vi "lorentzian from circle corners V7.vi"(6 "cursor bracket in":T1={"left"=2044.0881763527054, "right "=2126.7657992565055, "center"=2085.4269878046052, "window"=82.67762290380006, "cursors"=[], "relative"=0, "absolute"=0, "fixed vertical offset"=2421.6740576496672, "vertical offset"=2421.6740576496672, "skew"=2421.6740576496672, "default window frac"=2421.6740576496672, "kind"=enum."fancy", "skew.left"=2.0, "skew.right"=0.0, "Plot ref"=refnum, "wing order"=enum."back"}, 7 "update z(inf)":enum16{"update z(inf)", "do not update z(inf)"}(ring)=enum."do not update z(inf)", 8 "omega map rameters in":T7={"map method"=enum."less trivial", "2:window factor"=1, "left"=3.0, "right"=3.0, "omega"=3.0, "gamma"=3.0, "theta0"=3.0, "use points"=enum."decimated", "z(inf) method"=enum."median"}, 10 "parameters in: center detection":T6={"number of 2D grid points"=200, "# of points in pond"=93, "# of points in window"=4107, "decimation threshold"=1, "normalization factor"=0.005102552585135461, "pond scale factor "=3.0, "normalized z"=[], "decimated z"=[], "decimated omega"=[], "omega in window"=[], "z in window"=[], "data center"=-0.0014901433980738042-0.0014987103874714112i, "inverse"=[], "linear "=[], "omega around"=[], "phase around center"=[], "fit for phase around senter "=[], "three points"={[], []}, "max omega"=0.029014793, "min omega"=0.029014793, "dz/domega"=[]}, 11 "lorentzian in":T4={"A (VHz)"=-1.0311345636926572, "f (Hz)"=-1.0311345636926572, "G (Hz)"=-1.0311345636926572, "phi(rad)"=-1.0311345636926572, "Q"=-1.0311345636926572, "Norm  Ampl"=-1.0311345636926572, "bg (V)"=-1.0311345636926572+0.0i, "4corners"={"z (-pi/2)"=-1.0311345636926572+0.5736824521422934i, "z(inf)"=-0.5200164984937075+1.0975277942502903i, "z (pi/2)"=-1.0311345636926572+0.5736824521422934i, "z center"=-0.5136528600391839+0.580046090596817i, "z(0)"=-0.5200164984937075+1.0975277942502903i, "radius"=-1.0311345636926572}} {"bg (V)" format="%#9_9f"; "Q" format="%#9_9f"; "phi(rad)" format="%#9_9f"; "G (Hz)" format="%#9_9f"; "f (Hz)" format="%#9_9f"}) -> (0 "omega map parameters  out":T7={"map method"=enum."less trivial", "2:window factor"=1, "left"=3.0, "right"=3.0, "omega"=3.0, "gamma"=3.0, "theta0"=3.0, "use points"=enum."decimated", "z(inf) method"=enum."median"}, 2 "parameters out  : center detection":T6={"number of 2D grid points"=200, "# of points in pond"=93, "# of points in window"=4107, "decimation threshold"=1, "normalization factor"=0.005102552585135461, "pond scale factor "=3.0, "normalized z"=[], "decimated z"=[], "decimated omega"=[], "omega in window"=[], "z in window"=[], "data center"=-0.0014901433980738042-0.0014987103874714112i, "inverse"=[], "linear "=[], "omega around"=[], "phase around center"=[], "fit for phase around senter "=[], "three points"={[], []}, "max omega"=0.029014793, "min omega"=0.029014793, "dz/domega"=[]}, 3 "lorentzian out":T4={"A (VHz)"=-1.0311345636926572, "f (Hz)"=-1.0311345636926572, "G (Hz)"=-1.0311345636926572, "phi(rad)"=-1.0311345636926572, "Q"=-1.0311345636926572, "Norm  Ampl"=-1.0311345636926572, "bg (V)"=-1.0311345636926572+0.0i, "4corners"={"z (-pi/2)"=-1.0311345636926572+0.5736824521422934i, "z(inf)"=-0.5200164984937075+1.0975277942502903i, "z (pi/2)"=-1.0311345636926572+0.5736824521422934i, "z center"=-0.5136528600391839+0.580046090596817i, "z(0)"=-0.5200164984937075+1.0975277942502903i, "radius"=-1.0311345636926572}} {"bg (V)" format="%#9_9f"; "Q" format="%#9_9f"; "phi(rad)" format="%#9_9f"; "G (Hz)" format="%#9_9f"; "f (Hz)" format="%#9_9f"})   [LabVIEW 2018]
uses:
  lorentzian.ctl
  circle corners.ctl
  omega map parameters.ctl
  single fit parameters.ctl
  <vilib>/Utility/miscctls.llb/LVCursorListTypeDef.ctl
  cursor winow.ctl
  <vilib>/Utility/error.llb/Clear Errors.vi
  <vilib>/Analysis/baseanly.llb/Median.vi
  <vilib>/Analysis/baseanly.llb/Mean.vi
  <vilib>/Analysis/baseanly.llb/Mean (DBL).vi
  <vilib>/Analysis/2dsp.llb/Unwrap Phase.vi
  <vilib>/gmath/interp.llb/Interpolate 1D.vi
  peak -- fit function -- minus arctan.vi
  <vilib>/gmath/NumericalOptimization/Nonlinear Curve Fit.vi
  <vilib>/gmath/NumericalOptimization/Nonlinear Curve Fit LM.vi
  <vilib>/Analysis/6fits.llb/Linear Fit.vi
panel:
  in  "cursor window: fragment":T3
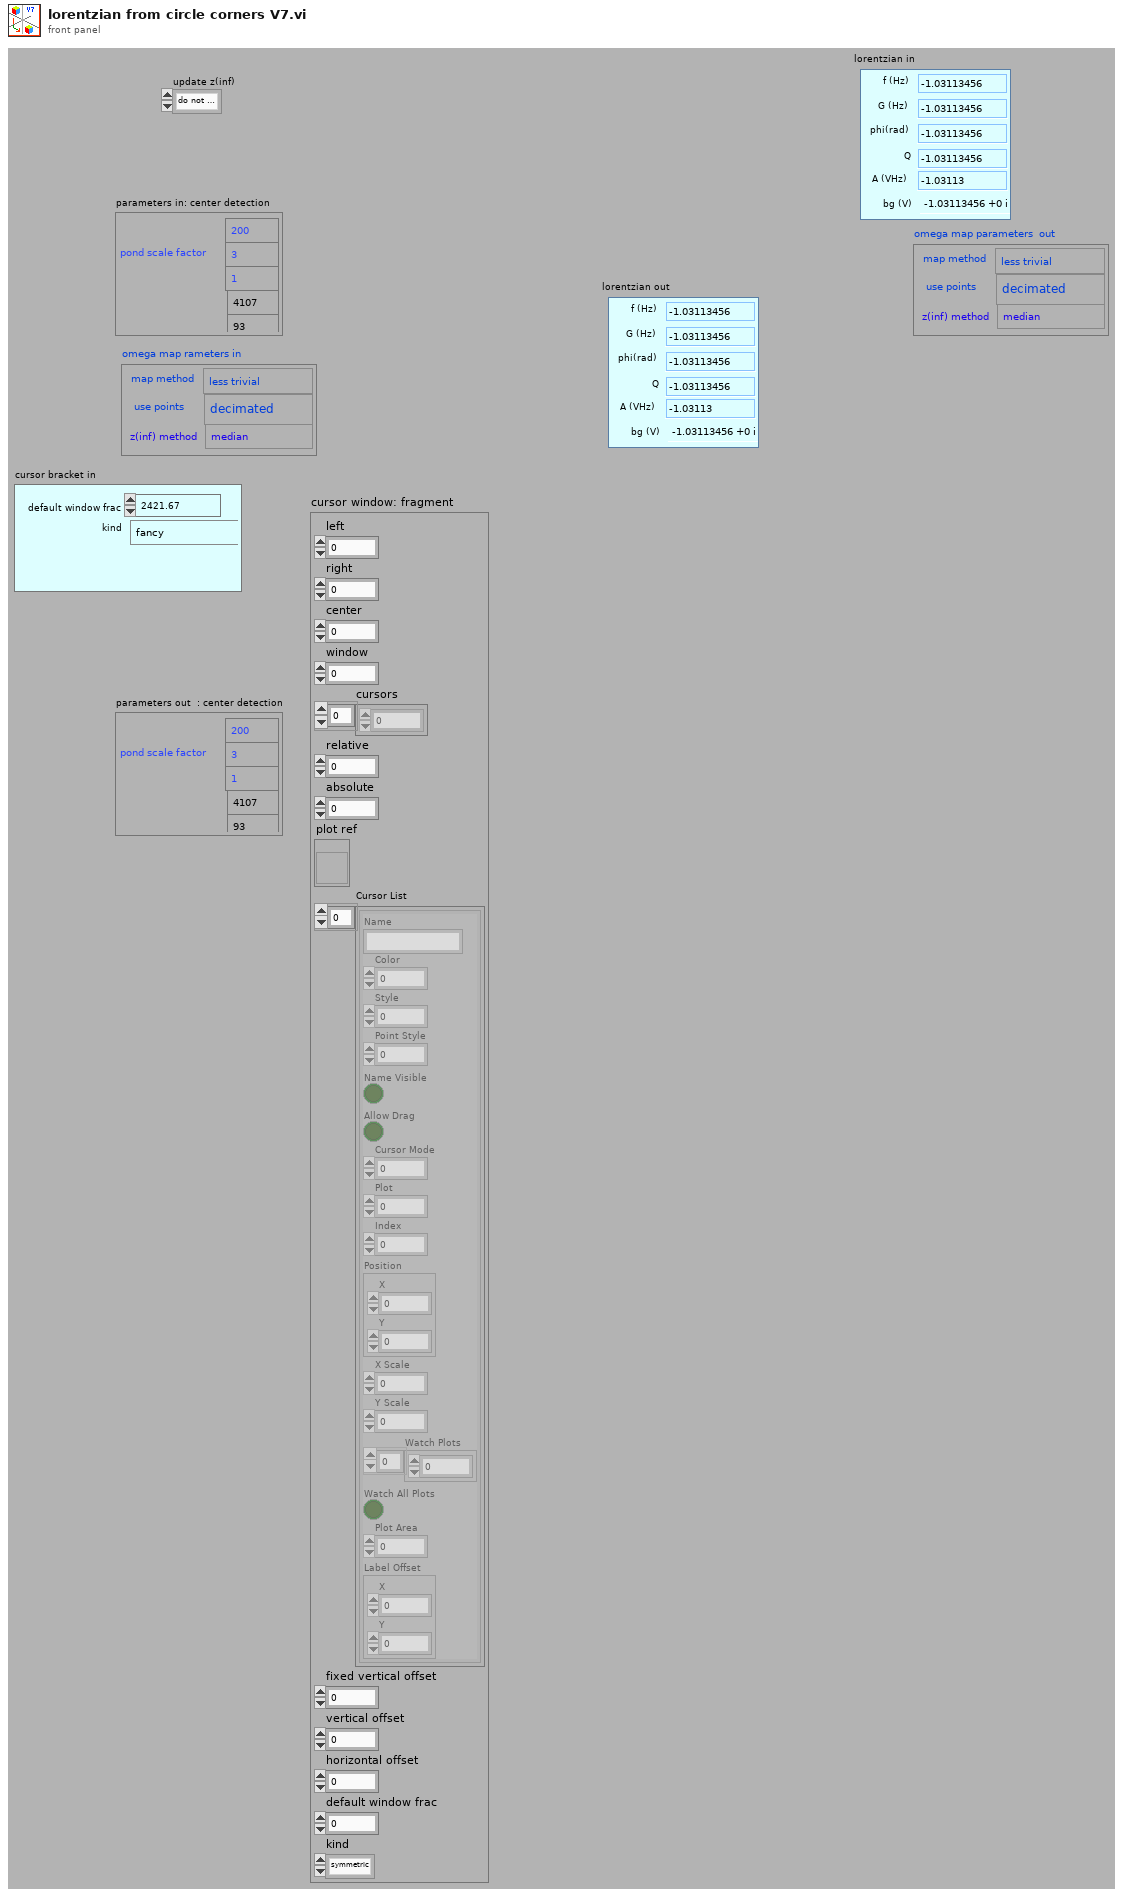
[diagram p1: front panel]
types:
  T1 = typedef "cursor winow.ctl" = cluster{"left":dbl, "right ":dbl, "center":dbl, "window":dbl, "cursors":i32[], "relative":i32, "absolute":i32, "fixed vertical offset":dbl, "vertical offset":dbl, "skew":dbl, "default window frac":dbl, "kind":enum16{"symmetric", "skewed", "fancy"}, "skew.left":dbl, "skew.right":dbl, "Plot ref":refnum<vi>, "wing order":enum16{"forw", "back"}}
  T2 = typedef "LVCursorListTypeDef.ctl" = cluster{"Name":string, "Color":u32, "Style":u8, "Point Style":u8, "Name Visible":bool, "Allow Drag":bool, "Cursor Mode":u32, "Plot":i32, "Index":i32, "Position":cluster{"X":dbl, "Y":dbl}, "X Scale":u32, "Y Scale":u32, "Watch Plots":i32[], "Watch All Plots":bool, "Plot Area":i32, "Label Offset":cluster{"X":dbl, "Y":dbl}}[]
  T3 = cluster{"left":dbl, "right ":dbl, "center":dbl, "window":dbl, "cursors":i32[], "relative":i32, "absolute":i32, "plot ref":refnum<vi>, "Cursor List":T2, "fixed vertical offset":dbl, "vertical offset":dbl, "horizontal offset":dbl, "default window frac":dbl, "kind":enum16{"symmetric", "skewed", "fancy"}}
  T4 = typedef "lorentzian.ctl" = cluster{"A (VHz)":dbl, "f (Hz)":dbl, "G (Hz)":dbl, "phi(rad)":dbl, "Q":dbl, "Norm  Ampl":dbl, "bg (V)":cdb, "4corners":T5}
  T5 = typedef "circle corners.ctl" = cluster{"z (-pi/2)":cdb, "z(inf)":cdb, "z (pi/2)":cdb, "z center":cdb, "z(0)":cdb, "radius":dbl}
  T6 = typedef "single fit parameters.ctl" = cluster{"number of 2D grid points":i32, "# of points in pond":i32, "# of points in window":i32, "decimation threshold":i32, "normalization factor":dbl, "pond scale factor ":dbl, "normalized z":cdb[], "decimated z":cdb[], "decimated omega":dbl[], "omega in window":dbl[], "z in window":cdb[], "data center":cdb, "inverse":cdb[], "linear ":cdb[], "omega around":dbl[], "phase around center":dbl[], "fit for phase around senter ":dbl[], "three points":cluster{dbl[], dbl[]}, "max omega":dbl, "min omega":dbl, "dz/domega":cdb[]}
  T7 = typedef "omega map parameters.ctl" = cluster{"map method":enum16{"simple", "less trivial", "around center", "geometry"}, "2:window factor":i32, "left":dbl, "right":dbl, "omega":dbl, "gamma":dbl, "theta0":dbl, "use points":enum16{"all in window", "decimated"}, "z(inf) method":enum16{"median", "method 2", "histogram"}}
  T8 = enum16{"simple", "less trivial", "around center", "geometry"}
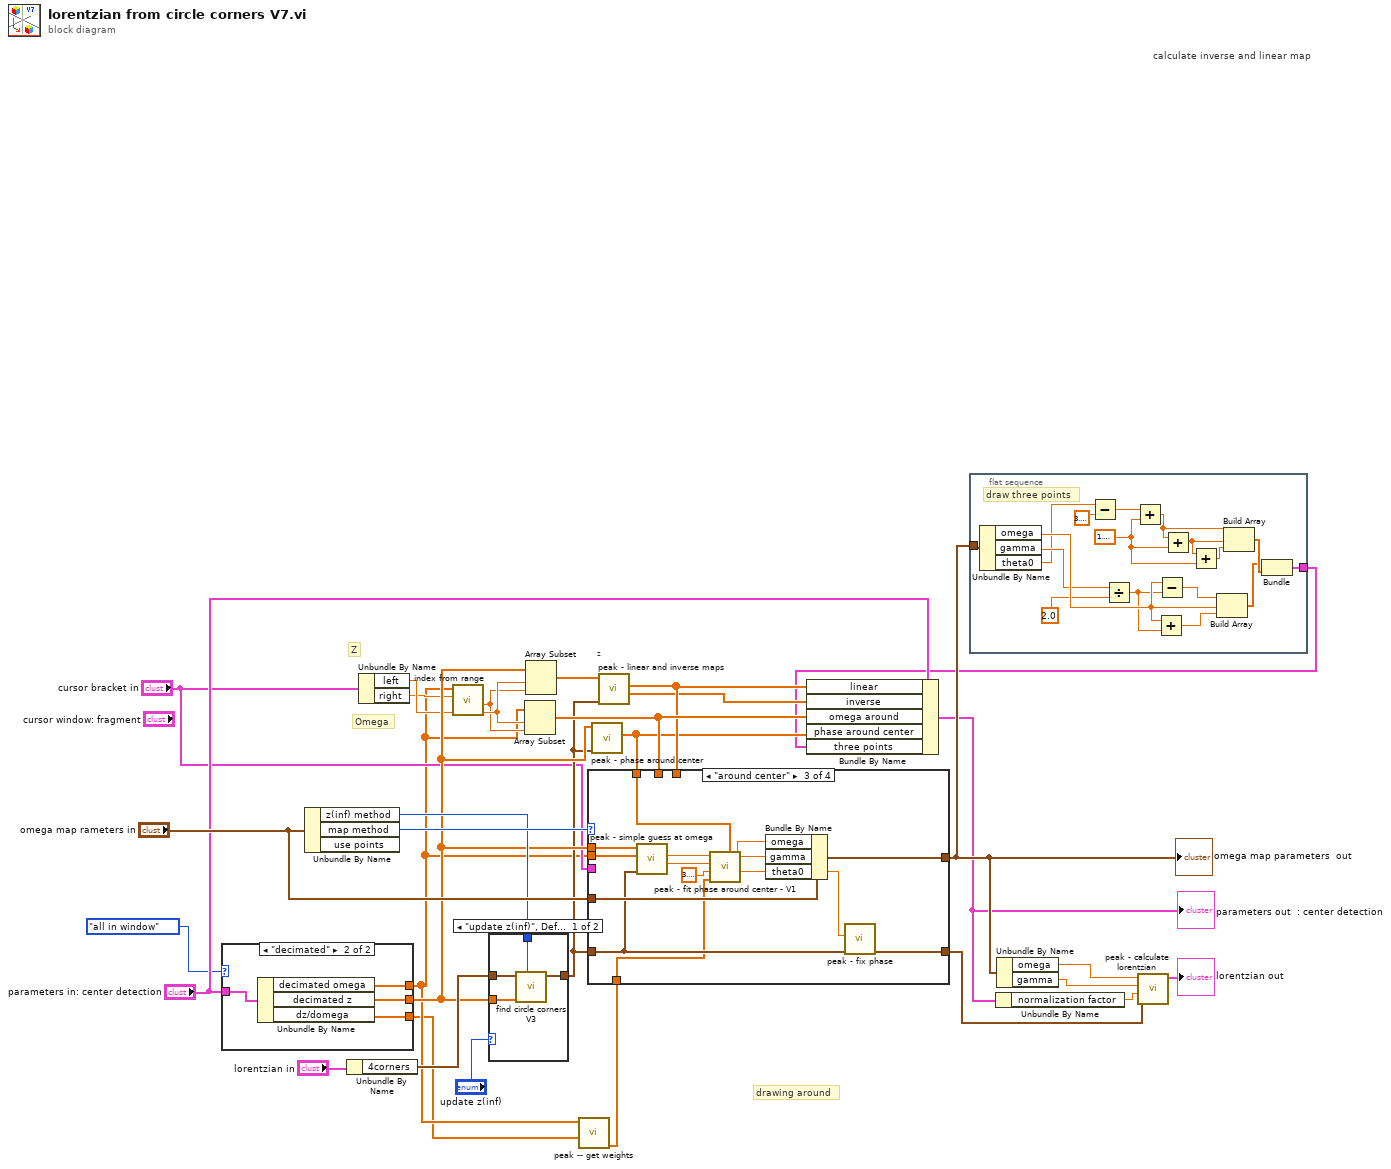
[diagram p0: block diagram]
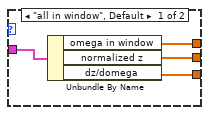
[diagram p3: hidden frame]
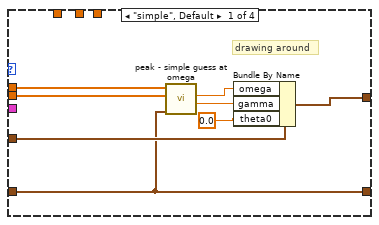
[diagram p4: hidden frame]
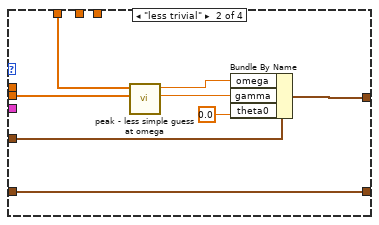
[diagram p5: hidden frame]
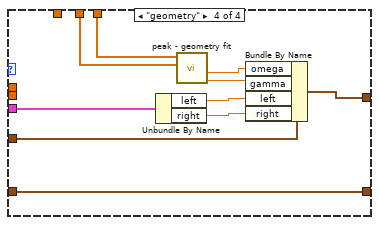
[diagram p6: hidden frame]
diagram:
  # "drawing around"
  # "z"
  # "Z"
  # "Omega"
  # "calculate inverse and linear map"
  n1 = case shown="\"decimated\"" enum16{"all in window", "decimated"}."all in window" ("use points") {
    tunnel: "parameters in: center detection" -> [w35 w39]
    tunnel: [w34 w38] -> w3
    tunnel: [w33 w37] -> w21
    tunnel: [w32 w36] -> w2
    frame "all in window", Default {
      n2 = Unbundle By Name(w35) -> ("omega in window"=w34:dbl[], "normalized z"=w33:cdb[], "dz/domega"=w32:cdb[])
    }
    frame "decimated" {
      n3 = Unbundle By Name(w39) -> ("decimated omega"=w38:dbl[], "decimated z"=w37:cdb[], "dz/domega"=w36:cdb[])
    }
  }
  n4 = Unbundle By Name("omega map rameters in") -> ("z(inf) method"=w24:enum16{"median", "method 2", "histogram"}, "map method"=w31:T8)  [unwired: 1 out]
  n5 = Unbundle By Name("lorentzian in") -> ("4corners"=w23:T5)
  n6 = Unbundle By Name("cursor bracket in") -> ("left"=w17:dbl, "right"=w16:dbl)
  n7 = call "index from range.vi"("left"=w17, "right"=w16, "omega"=w3) -> ("left index"=w15:dbl, "length"=w14:dbl)  [unwired: 6 in, 1 out]
  n8 = case shown="\"update z(inf)\", Default" "update z(inf)" {
    tunnel: [w42 w44] -> w20
    tunnel: w23 -> [w43 w44]
    tunnel: w21 -> [w41 _]
    tunnel: w24 -> [w40 _]
    frame "update z(inf)", Default {
      n9 = call "find circle corners V3.vi"("method"=w40, "z"=w41, "circle corners in"=w43) -> ("circle corners out"=w42:T5)  [unwired: 8 in]
    }
    frame "do not update z(inf)" {
    }
  }
  n10 = Array Subset(array=w3, index=w15, length=w14) -> (w28:dbl[])
  n11 = Array Subset(array=w21, index=w15, length=w14) -> (w19:cdb[])
  n12 = call "peak -- get weights.vi"("dz/domega"=w2, "omega"=w3) -> ("weights"=w1:dbl[])  [unwired: 8 in, 1 out]
  n13 = call "peak - phase around center.vi"("4corners"=w20, "z"=w21) -> ("Unwrapped Phase"=w8:dbl[])  [unwired: 9 in]
  n14 = call "peak - linear and inverse maps.vi"("4corners"=w20, "Z"=w19) -> ("inverse"=w18:cdb[], "linear"=w27:cdb[])  [unwired: 8 in]
  n15 = case shown="\"around center\"" w31 {
    tunnel: w20 -> [w49 w58 w71 w80]
    tunnel: w21 -> [w48 _ w72 _]
    tunnel: w3 -> [w47 w55 w63 _]
    tunnel: "omega map rameters in" -> [w51 w60 w73 w77]
    tunnel: [w50 w59 w74 w84] -> w10
    tunnel: "cursor bracket in" -> [_ _ _ w83]
    tunnel: w28 -> [_ _ _ w82]
    tunnel: w27 -> [_ _ _ w81]
    tunnel: w8 -> [_ w56 w62 _]
    tunnel: [w49 w58 w70 w80] -> w25
    tunnel: w1 -> [_ _ w61 _]
    frame "simple", Default {
      # "drawing around"
      n16 = call "peak - simple guess at omega.vi"("4corners"=w49, "omega"=w47, "z"=w48) -> ("guess at gamma"=w45:dbl, "guess at omega"=w46:dbl)  [unwired: 7 in]
      n17 = Bundle By Name(cluster=w51, "omega"=w46, "gamma"=w45, "theta0"=0.0 ("phi0")) -> (w50:T7)
    }
    frame "less trivial" {
      n18 = call "peak - less simple guess at omega.vi"("omega"=w55, "Unwrapped Phase"=w56) -> ("gamma guess"=w54:dbl, "omega guess"=w53:dbl)  [unwired: 8 in]
      n19 = Bundle By Name(cluster=w60, "omega"=w53, "gamma"=w54, "theta0"=0.0 ("phi0")) -> (w59:T7)
    }
    frame "around center" {
      n20 = call "peak - simple guess at omega.vi"("4corners"=w71, "omega"=w63, "z"=w72) -> ("guess at gamma"=w68:dbl, "guess at omega"=w69:dbl)  [unwired: 7 in]
      n21 = call "peak - fit phase around center - V1.vi"("Phase"=w62, "omega"=w63, "weights"=w61, "guess at theta"=3.141592653589793, "guess at gamma"=w68, "guess at omega"=w69) -> ("fit for theta"=w64:dbl, "fit for gamma"=w65:dbl, "fit for omega"=w66:dbl)  [unwired: 3 in]
      n22 = Bundle By Name(cluster=w73, "omega"=w66, "gamma"=w65, "theta0"=w64) -> (w74:T7)
      n23 = call "peak - fix phase.vi"("4corners"=w71, "correct phase"=w64) -> ("4corners out"=w70:T5)  [unwired: 9 in]
    }
    frame "geometry" {
      n24 = Unbundle By Name(w83) -> ("left"=w79:dbl, "right"=w78:dbl)
      n25 = call "peak - geometry fit.vi"("omega"=w82, "linear z"=w81) -> ("gamma"=w75:dbl, "omega"=w76:dbl)  [unwired: 8 in]
      n26 = Bundle By Name(cluster=w77, "omega"=w76, "gamma"=w75, "left"=w79, "right"=w78) -> (w84:T7)
    }
  }
  "omega map parameters  out" <- w10
  n27 = Bundle By Name(cluster="parameters in: center detection", "linear"=w27, "inverse"=w18, "omega around"=w28, "phase around center"=w8, "three points"=w7) -> (w6:T6)
  "parameters out  : center detection" <- w6
  n28 = flat-sequence {
    tunnel: w10 -> [w101]
    tunnel: [w97] -> w7
    frame #0 {
      w89 = 1.5707963267948966
      # "draw three points"
      n29 = Unbundle By Name(w101) -> ("omega"=w100:dbl, "gamma"=w99:dbl, "theta0"=w98:dbl)
      n30 = Subtract(x=w98, y=3.141592653589793) -> (x-y=w85:dbl)
      n31 = Divide(x=w99, y=2.0) -> (x/y=w87:dbl)
      n32 = Add(x=w85, y=w89) -> (x+y=w90:dbl)
      n33 = Add(x=w100, y=w87) -> (x+y=w91:dbl)
      n34 = Subtract(x=w100, y=w87) -> (x-y=w92:dbl)
      n35 = Add(x=w90, y=w89) -> (x+y=w96:dbl)
      n36 = Add(x=w96, y=w89) -> (x+y=w95:dbl)
      n37 = Build Array(w92, w100, w91) -> (w93:dbl[])
      n38 = Build Array(w90, w96, w95) -> (w94:dbl[])
      n39 = Bundle(w93, w94) -> (w97:cluster{dbl[], dbl[]})  [unwired: 1 in]
    }
  }
  n40 = Unbundle By Name(w6) -> ("normalization factor"=w13:dbl)
  n41 = Unbundle By Name(w10) -> ("omega"=w12:dbl, "gamma"=w11:dbl)
  n42 = call "peak - calculate lorentzian.vi"("4corners"=w25, "normalization factor"=w13, "gamma"=w11, "omega"=w12) -> ("lorentzian out"=→"lorentzian out":T4)  [unwired: 7 in]
